vi "Set Speaker Switch.vi"(8 "error in":errorcluster, 10 "State":bool, 11 "PAS in":refnum<class "PAS.lvclass">) -> (0 "error out":errorcluster, 3 "PAS out":refnum<class "PAS.lvclass">)   [LabVIEW 2014, in "PAS Library.lvlib" / "PAS.lvclass"]
uses:
  PAS.lvclass
  Data/Main/PAS Data.lvclass
  Instrument/Instrument.lvclass/Instrument.ctl
  PAS.lvclass/PAS.ctl
  Instrument/Read Data.vi
  Instrument/Write Data.vi
  Data/Data.lvclass
  Switch/Switch.lvclass
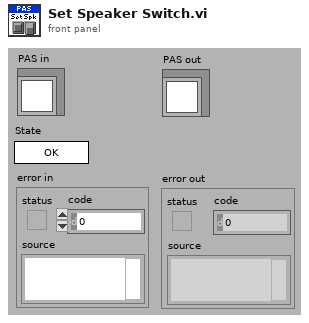
[diagram p1: front panel]
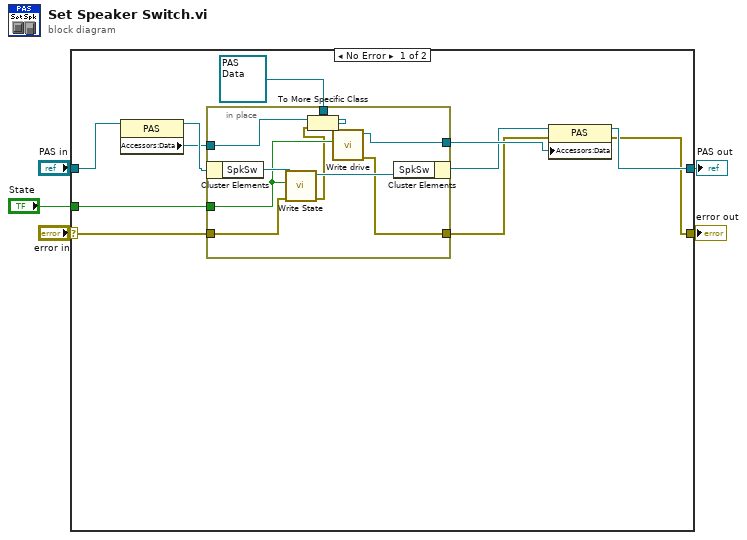
[diagram p0: block diagram]
diagram:
  n1 = case shown="No Error" "error in" {
    selector: "error in" -> [w16 w29]
    tunnel: [w6 w29] -> w4
    tunnel: [w8 w28] -> w2
    tunnel: "PAS in" -> [w13 w28]
    tunnel: "State" -> [w15 _]
    frame No Error {
      n2 = property class="PAS"(reference=w13) -> (reference out=w12:refnum<class "PAS.lvclass">, "Accessors:Data"=w11:refnum<class "Data.lvclass">)  [unwired: 1 in, 1 out]
      n3 = in-place {
        in-place-border: w16 -> [w25]
        in-place-border: [w24] -> w7
        in-place-border: w15 -> [w23]
        in-place-border: refnum<class "PAS Data.lvclass"> refnum ("PAS Data") -> [w22]
        in-place-border: w11 -> [w19]
        in-place-border: [w18] -> w10
        n4 = in-place-cluster #1(w12) -> ("SpkSw"=w27:refnum<class "Switch.lvclass">)
        n5 = call-dynamic "Write State.vi"("error in"=w25, "State"=w23, "Switch in"=w27) -> ("error out"=w20:errorcluster, "Switch out"=w26:refnum<class "Switch.lvclass">)  [unwired: 7 in]
        n6 = To More Specific Class(target class=w22, reference=w19, error in=w20) -> (specific class reference=w21:refnum<class "PAS Data.lvclass">, error out=w17:errorcluster)
        n7 = call "Write drive.vi"("error in"=w17, "drive"=w23, "PAS Data in"=w21) -> ("error out"=w24:errorcluster, "PAS Data out"=w18:refnum<class "PAS Data.lvclass">)  [unwired: 7 in]
        n8 = in-place-cluster #1("SpkSw"=w26) -> (w9:refnum<class "PAS.lvclass">)
      }
      n9 = property class="PAS"(reference=w9, error in=w7, "Accessors:Data"=w10) -> (reference out=w8:refnum<class "PAS.lvclass">, error out=w6:errorcluster)
    }
    frame Error {
    }
  }
  "error out" <- w4
  "PAS out" <- w2
